vi "SVPO RMS Level.vi"   [LabVIEW 2017, in "SoundVib_VibrationLevel.lvlib"]
doc: "Computes the root-mean-square (RMS) level of scaled time waveform signals and scaled array signals. <B>scaled signal [EU]</B> should have a zero DC component. You can attenuate the DC component with hardware AC-coupling filters and with software high-pass filters. Use this VI on embedded targets that have limited computational resources. Wire data to the <B>scaled signal [EU]</B> input to determine the polymorphic instance to use or manually select the instance."
uses:
  <vilib>/addons/Sound and Vibration/svt_Level/SoundVib_VibrationLevel.lvlib
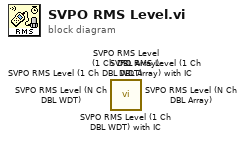
[diagram p0: block diagram]
diagram:
  n1 = call <vilib>:"SVPO RMS Level (1 Ch DBL WDT) with IC.vi"() -> ()  [unwired: 8 in, 4 out]
  n2 = call <vilib>:"SVPO RMS Level (1 Ch DBL Array) with IC.vi"() -> ()  [unwired: 9 in, 3 out]
  n3 = call <vilib>:"SVPO RMS Level (N Ch DBL WDT).vi"() -> ()  [unwired: 9 in, 3 out]
  n4 = call <vilib>:"SVPO RMS Level (N Ch DBL Array).vi"() -> ()  [unwired: 10 in, 2 out]
  n5 = call <vilib>:"SVPO RMS Level (1 Ch DBL WDT).vi"() -> ()  [unwired: 9 in, 3 out]
  n6 = call <vilib>:"SVPO RMS Level (1 Ch DBL Array).vi"() -> ()  [unwired: 10 in, 2 out]
